vi "btc-private-to-address.vi"(8 "error in (no error)":cluster{"状态":bool, "代码":i32, "源":string} caption="错误输入（无错误）", 11 "私钥输入":string="a9ddf02d9a749a49db0c29eef84fdbcf82e7f3e3c63d1c989c2118296439e9da") -> (0 "error out":cluster{"状态":bool, "代码":i32, "源":string} caption="错误输出", 1 "非压缩地址":string, 3 "压缩地址":string)   [LabVIEW 2020]
uses:
  C:/Program Files (x86)/National Instruments/LabVIEW 2020/examples/Connectivity/Python/support/PythonVersionsEnum.ctl
panel:
  in  "Python版本":T1=enum."3.6"
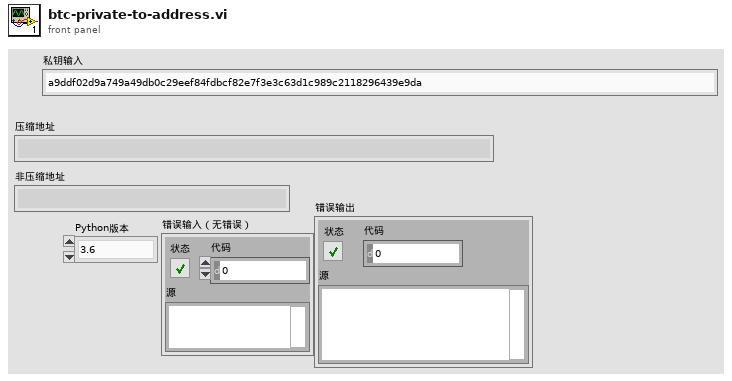
[diagram p1: front panel]
types:
  T1 = typedef "PythonVersionsEnum.ctl" = enum16{"2.7", "3.6"}
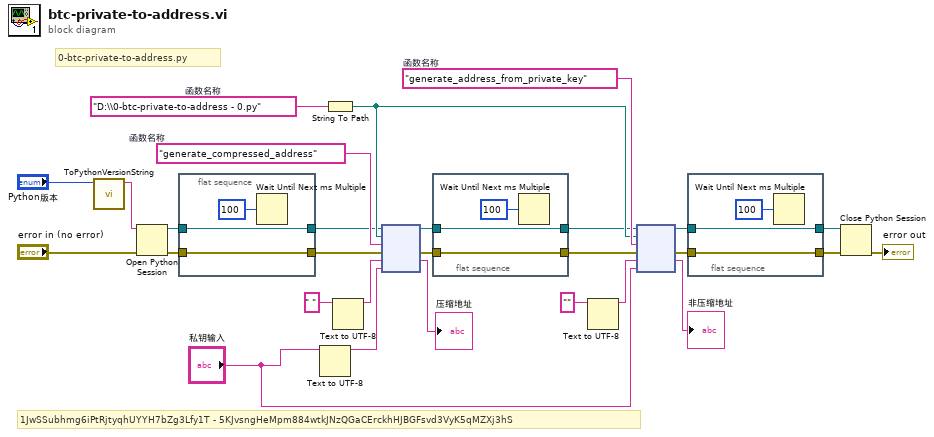
[diagram p0: block diagram]
diagram:
  w22 = "generate_address_from_private_key"  # 函数名称
  w24 = "generate_compressed_address"  # 函数名称
  w25 = "D:\\0-btc-private-to-address - 0.py"  # 函数名称
  # "0-btc-private-to-address.py"
  # "1JwSSubhmg6iPtRjtyqhUYYH7bZg3Lfy1T - 5KJvsngHeMpm884wtkJNzQGaCErckhHJBGFsvd3VyK5qMZXj3hS"
  n1 = call "ToPythonVersionString.vi"("Python版本"="Python版本") -> ("python版本字符串"=w28:string)  [unwired: 10 in]
  n2 = Open Python Session(python version=w28, 3:"error in (no error)") -> (session out=w17:refnum<k35>, error out=w7:errorcluster)  [unwired: 1 in]
  n3 = flat-sequence {
    tunnel: w17 -> [w30]
    tunnel: [w30] -> w16
    tunnel: [w29] -> w6
    tunnel: w7 -> [w29]
    frame #0 {
      n4 = Wait Until Next ms Multiple(millisecond multiple=u32 100 ("毫秒倍数")) -> ()  [unwired: 1 out]
    }
  }
  n5 = Text to UTF-8(11:"私钥输入") -> (3:w23:string)  [unwired: 2 in, 1 out]
  n6 = String To Path(string=w25) -> (path=w18:path)
  n7 = Text to UTF-8(11:" ") -> (3:w21:string)  [unwired: 2 in, 1 out]
  n8 = node(w16, w18, w24, w6, w21, w23) -> (w15:refnum<k35>, w5:errorcluster, →"压缩地址":string)  [unwired: 1 in, 2 out]
  n9 = flat-sequence {
    tunnel: w15 -> [w33]
    tunnel: [w33] -> w14
    tunnel: [w32] -> w4
    tunnel: w5 -> [w32]
    frame #0 {
      n10 = Wait Until Next ms Multiple(millisecond multiple=u32 100 ("毫秒倍数")) -> ()  [unwired: 1 out]
    }
  }
  n11 = Text to UTF-8(11:"") -> (3:w8:string)  [unwired: 2 in, 1 out]
  n12 = node(w14, w18, w22, w4, w8, "私钥输入") -> (w11:refnum<k35>, w2:errorcluster, →"非压缩地址":string)  [unwired: 1 in, 2 out]
  n13 = flat-sequence {
    tunnel: [w36] -> w10
    tunnel: w11 -> [w36]
    tunnel: [w35] -> w3
    tunnel: w2 -> [w35]
    frame #0 {
      n14 = Wait Until Next ms Multiple(millisecond multiple=u32 100 ("毫秒倍数")) -> ()  [unwired: 1 out]
    }
  }
  n15 = Close Python Session(session in=w10, error in=w3) -> (11:→"error out":errorcluster)
